vi "FeedbackDecode_20200902.vi"() -> ()   [LabVIEW 2016] (continued)
                n759 = Format Into String(w469) -> (resulting string=w459:string)  [unwired: 3 in, 1 out]
                n760 = Concatenate Strings("ExcludeSE:SS.EventID=" ("string"), w459) -> (w468:string)
                n761 = call-poly "FeedbackDecode_VariablesToString.vi"("Format"="%0.0f", "ValueIn"=w463, "FieldName"="NIPTime" ("Key Word")) -> ("StringOut"=w460:string)  [unwired: 4 in]
                n762 = local read "EventParamsFID"() -> (w466:refnum<file>)
                n763 = local read "DecodeClust"() -> (w472:T5)
                n764 = Concatenate Strings(w468, ";SS.ExcludeSE=1;" ("EventStr"), w460) -> (w465:string)
                n765 = call "FeedbackDecode_WriteTextEOL.vi"("text"=w465, "refnum in"=w466) -> ()  [unwired: 8 in, 2 out]
                n766 = Bundle By Name(cluster=w472, "EventStr"=w465) -> (w464:T5)
                n767 = call "FeedbackDecode_MLComCtrl.vi"("DecodeClustIn"=w464, "Mode"=T19."SendEvent") -> ()  [unwired: 6 in, 4 out]
              }
            }
          }
          event Value Change {
            n768 = event-data() -> ("NewVal"=w474:bool)  [unwired: 1 in, 5 out]
            n769 = case shown="True" w474 {
              frame False {
                n770 = local read "LoopCnt"() -> (w485:u64)
                n771 = local read "NIPTime"() -> (w479:dbl)
                n772 = Format Into String(w485) -> (resulting string=w475:string)  [unwired: 3 in, 1 out]
                n773 = Concatenate Strings("StopAcqCAR:SS.EventID=" ("string"), w475) -> (w484:string)
                n774 = local read "EventParamsFID"() -> (w482:refnum<file>)
                n775 = call-poly "FeedbackDecode_VariablesToString.vi"("Format"="%0.0f", "ValueIn"=w479, "FieldName"="NIPTime" ("Key Word")) -> ("StringOut"=w476:string)  [unwired: 4 in]
                n776 = local read "DecodeClust"() -> (w488:T5)
                n777 = Concatenate Strings(w484, ";SS.AcqCAR=0;" ("EventStr"), w476) -> (w481:string)
                n778 = call "FeedbackDecode_WriteTextEOL.vi"("text"=w481, "refnum in"=w482) -> ()  [unwired: 8 in, 2 out]
                n779 = Bundle By Name(cluster=w488, "EventStr"=w481) -> (w480:T5)
                n780 = call "FeedbackDecode_MLComCtrl.vi"("DecodeClustIn"=w480, "Mode"=T19."SendEvent") -> ()  [unwired: 6 in, 4 out]
              }
              frame True {
                n781 = local read "LoopCnt"() -> (w499:u64)
                n782 = local read "NIPTime"() -> (w493:dbl)
                n783 = Format Into String(w499) -> (resulting string=w489:string)  [unwired: 3 in, 1 out]
                n784 = call-poly "FeedbackDecode_VariablesToString.vi"("Format"="%0.0f", "ValueIn"=w493, "FieldName"="NIPTime" ("Key Word")) -> ("StringOut"=w490:string)  [unwired: 4 in]
                n785 = Concatenate Strings("StartAcqCAR:SS.EventID=" ("string"), w489) -> (w498:string)
                n786 = local read "EventParamsFID"() -> (w496:refnum<file>)
                n787 = local read "DecodeClust"() -> (w502:T5)
                n788 = Concatenate Strings(w498, ";SS.AcqCAR=1;" ("EventStr"), w490) -> (w495:string)
                n789 = call "FeedbackDecode_WriteTextEOL.vi"("text"=w495, "refnum in"=w496) -> ()  [unwired: 8 in, 2 out]
                n790 = Bundle By Name(cluster=w502, "EventStr"=w495) -> (w494:T5)
                n791 = call "FeedbackDecode_MLComCtrl.vi"("DecodeClustIn"=w494, "Mode"=T19."SendEvent") -> ()  [unwired: 6 in, 4 out]
              }
            }
          }
          event Value Change {
            n792 = event-data() -> ("NewVal"=w504:bool)  [unwired: 1 in, 5 out]
            n793 = case shown="True" w504 {
              frame False {
              }
              frame True {
                n794 = stacked-sequence {
                  frame #0 {
                    n795 = local read "DecodeClust"() -> (w522:T5)
                    n796 = call "FeedbackDecode_MLComCtrl.vi"("DecodeClustIn"=w522, "Mode"=T19."BuildKalmanStr") -> ("DecodeClustOut"=w521:T5)  [unwired: 6 in, 3 out]
                    n797 = Unbundle By Name(w521) -> ("EventStr"=w529:string, "KalmanType"=w510:T44, "KDFFile"=w514:string)
                    n798 = local read "LoopCnt"() -> (w525:u64)
                    n799 = local read "NIPTime"() -> (w519:dbl)
                    n800 = Format Into String(format string="%s", w510) -> (resulting string=w507:string)  [unwired: 2 in, 1 out]
                    n801 = Format Into String(w525) -> (resulting string=w505:string)  [unwired: 3 in, 1 out]
                    n802 = call-poly "FeedbackDecode_VariablesToString.vi"("ValueIn"=w514, "FieldName"="KDFFile") -> ("StringOut"=w513:string)  [unwired: 5 in]
                    n803 = call-poly "FeedbackDecode_VariablesToString.vi"("Format"="%0.0f", "ValueIn"=w519, "FieldName"="NIPTime" ("Key Word")) -> ("StringOut"=w512:string)  [unwired: 4 in]
                    n804 = Concatenate Strings("ApplyTraining:SS.EventID=" ("string"), w505) -> (w524:string)
                    n805 = Concatenate Strings(w524, ";", w529) -> (w516:string)
                    n806 = local read "EventParamsFID"() -> (w523:refnum<file>)
                    n807 = Bundle By Name(cluster=w521, "EventStr"=w516) -> (w520:T5)
                    n808 = Concatenate Strings(w516, "SS.DecodeType='" ("FieldName"), w507, "';" ("string"), w513, w512) -> (w511:string)
                    n809 = call "FeedbackDecode_WriteTextEOL.vi"("text"=w511, "refnum in"=w523) -> ()  [unwired: 8 in, 2 out]
                    n810 = call "FeedbackDecode_MLComCtrl.vi"("DecodeClustIn"=w520, "Mode"=T19."SendEvent") -> ()  [unwired: 6 in, 4 out]
                  }
                  frame #1 {
                    n811 = property on="KinSrc" class="Enum (strict)"("Val(Sgnl)"=enum16{"Off", "Training", "Decode", "COB"}."Decode" ("Value (Signaling)")) -> ()  [unwired: 2 in, 2 out]
                  }
                }
              }
            }
          }
          event Value Change {
            n812 = event-data() -> ("NewVal"=w532:bool)  [unwired: 1 in, 5 out]
            n813 = case shown="True" w532 {
              frame False {
                n814 = local read "LoopCnt"() -> (w544:u64)
                n815 = local read "NIPTime"() -> (w538:dbl)
                n816 = Format Into String(w544) -> (resulting string=w534:string)  [unwired: 3 in, 1 out]
                n817 = call-poly "FeedbackDecode_VariablesToString.vi"("Format"="%0.0f", "ValueIn"=w538, "FieldName"="NIPTime" ("Key Word")) -> ("StringOut"=w535:string)  [unwired: 4 in]
                n818 = Concatenate Strings("DisableBaseline:SS.EventID=" ("string"), w534) -> (w543:string)
                n819 = local read "EventParamsFID"() -> (w541:refnum<file>)
                n820 = local read "DecodeClust"() -> (w547:T5)
                n821 = Concatenate Strings(w543, ";SS.ApplyBaseline=0;" ("EventStr"), w535) -> (w540:string)
                n822 = call "FeedbackDecode_WriteTextEOL.vi"("text"=w540, "refnum in"=w541) -> ()  [unwired: 8 in, 2 out]
                n823 = Bundle By Name(cluster=w547, "EventStr"=w540) -> (w539:T5)
                n824 = call "FeedbackDecode_MLComCtrl.vi"("DecodeClustIn"=w539, "Mode"=T19."SendEvent") -> ()  [unwired: 6 in, 4 out]
              }
              frame True {
                n825 = local read "LoopCnt"() -> (w558:u64)
                n826 = local read "NIPTime"() -> (w552:dbl)
                n827 = Format Into String(w558) -> (resulting string=w548:string)  [unwired: 3 in, 1 out]
                n828 = Concatenate Strings("EnableBaseline:SS.EventID=" ("string"), w548) -> (w557:string)
                n829 = local read "EventParamsFID"() -> (w555:refnum<file>)
                n830 = call-poly "FeedbackDecode_VariablesToString.vi"("Format"="%0.0f", "ValueIn"=w552, "FieldName"="NIPTime" ("Key Word")) -> ("StringOut"=w549:string)  [unwired: 4 in]
                n831 = local read "DecodeClust"() -> (w561:T5)
                n832 = Concatenate Strings(w557, ";SS.ApplyBaseline=1;" ("EventStr"), w549) -> (w554:string)
                n833 = call "FeedbackDecode_WriteTextEOL.vi"("text"=w554, "refnum in"=w555) -> ()  [unwired: 8 in, 2 out]
                n834 = Bundle By Name(cluster=w561, "EventStr"=w554) -> (w553:T5)
                n835 = call "FeedbackDecode_MLComCtrl.vi"("DecodeClustIn"=w553, "Mode"=T19."SendEvent") -> ()  [unwired: 6 in, 4 out]
              }
            }
          }
          event Value Change {
            n836 = event-data() -> ("NewVal"=w562:bool)  [unwired: 1 in, 5 out]
            n837 = case shown="True" w562 {
              frame False {
                n838 = disable-structure shown="Disabled" {
                  frame Disabled {
                    n839 = local read "LoopCnt"() -> (w574:u64)
                    n840 = local read "NIPTime"() -> (w568:dbl)
                    n841 = Format Into String(w574) -> (resulting string=w564:string)  [unwired: 3 in, 1 out]
                    n842 = call-poly "FeedbackDecode_VariablesToString.vi"("Format"="%0.0f", "ValueIn"=w568, "FieldName"="NIPTime" ("Key Word")) -> ("StringOut"=w565:string)  [unwired: 4 in]
                    n843 = Concatenate Strings("DisableBaseline:SS.EventID=" ("string"), w564) -> (w573:string)
                    n844 = local read "EventParamsFID"() -> (w571:refnum<file>)
                    n845 = local read "DecodeClust"() -> (w577:T5)
                    n846 = Concatenate Strings(w573, ";SS.ApplyBaseline=0;" ("EventStr"), w565) -> (w570:string)
                    n847 = call "FeedbackDecode_WriteTextEOL.vi"("text"=w570, "refnum in"=w571) -> ()  [unwired: 8 in, 2 out]
                    n848 = Bundle By Name(cluster=w577, "EventStr"=w570) -> (w569:T5)
                    n849 = call "FeedbackDecode_MLComCtrl.vi"("DecodeClustIn"=w569, "Mode"=T19."SendEvent") -> ()  [unwired: 6 in, 4 out]
                  }
                  frame Enabled {
                  }
                }
              }
              frame True {
                n850 = local read "LoopCnt"() -> (w588:u64)
                n851 = local read "NIPTime"() -> (w582:dbl)
                n852 = Format Into String(w588) -> (resulting string=w578:string)  [unwired: 3 in, 1 out]
                n853 = Concatenate Strings("ExportTraining:SS.EventID=" ("string"), w578) -> (w587:string)
                n854 = local read "EventParamsFID"() -> (w585:refnum<file>)
                n855 = call-poly "FeedbackDecode_VariablesToString.vi"("Format"="%0.0f", "ValueIn"=w582, "FieldName"="NIPTime" ("Key Word")) -> ("StringOut"=w579:string)  [unwired: 4 in]
                n856 = local read "DecodeClust"() -> (w591:T5)
                n857 = Concatenate Strings(w587, ";SS.ExportTraining=1;" ("EventStr"), w579) -> (w584:string)
                n858 = call "FeedbackDecode_WriteTextEOL.vi"("text"=w584, "refnum in"=w585) -> ()  [unwired: 8 in, 2 out]
                n859 = Bundle By Name(cluster=w591, "EventStr"=w584) -> (w583:T5)
                n860 = call "FeedbackDecode_MLComCtrl.vi"("DecodeClustIn"=w583, "Mode"=T19."SendEvent") -> ()  [unwired: 6 in, 4 out]
              }
            }
          }
          event Value Change {
            n861 = event-data() -> ("NewVal"=w592:bool)  [unwired: 1 in, 5 out]
            n862 = case shown="True" w592 {
              frame False {
                n863 = local read "LoopCnt"() -> (w604:u64)
                n864 = local read "NIPTime"() -> (w598:dbl)
                n865 = Format Into String(w604) -> (resulting string=w594:string)  [unwired: 3 in, 1 out]
                n866 = call-poly "FeedbackDecode_VariablesToString.vi"("Format"="%0.0f", "ValueIn"=w598, "FieldName"="NIPTime" ("Key Word")) -> ("StringOut"=w595:string)  [unwired: 4 in]
                n867 = Concatenate Strings("LatchingFilter:SS.EventID=" ("string"), w594) -> (w603:string)
                n868 = local read "EventParamsFID"() -> (w601:refnum<file>)
                n869 = local read "DecodeClust"() -> (w607:T5)
                n870 = Concatenate Strings(w603, ";SS.LatchingFilter=0;" ("EventStr"), w595) -> (w600:string)
                n871 = call "FeedbackDecode_WriteTextEOL.vi"("text"=w600, "refnum in"=w601) -> ()  [unwired: 8 in, 2 out]
                n872 = Bundle By Name(cluster=w607, "EventStr"=w600) -> (w599:T5)
                n873 = call "FeedbackDecode_MLComCtrl.vi"("DecodeClustIn"=w599, "Mode"=T19."SendEvent") -> ()  [unwired: 6 in, 4 out]
              }
              frame True {
                n874 = local read "LoopCnt"() -> (w618:u64)
                n875 = local read "NIPTime"() -> (w612:dbl)
                n876 = Format Into String(w618) -> (resulting string=w608:string)  [unwired: 3 in, 1 out]
                n877 = Concatenate Strings("LatchingFilter:SS.EventID=" ("string"), w608) -> (w617:string)
                n878 = local read "EventParamsFID"() -> (w615:refnum<file>)
                n879 = call-poly "FeedbackDecode_VariablesToString.vi"("Format"="%0.0f", "ValueIn"=w612, "FieldName"="NIPTime" ("Key Word")) -> ("StringOut"=w609:string)  [unwired: 4 in]
                n880 = local read "DecodeClust"() -> (w621:T5)
                n881 = Concatenate Strings(w617, ";SS.LatchingFilter=1;" ("EventStr"), w609) -> (w614:string)
                n882 = call "FeedbackDecode_WriteTextEOL.vi"("text"=w614, "refnum in"=w615) -> ()  [unwired: 8 in, 2 out]
                n883 = Bundle By Name(cluster=w621, "EventStr"=w614) -> (w613:T5)
                n884 = call "FeedbackDecode_MLComCtrl.vi"("DecodeClustIn"=w613, "Mode"=T19."SendEvent") -> ()  [unwired: 6 in, 4 out]
              }
            }
          }
          event Value Change {
            n885 = event-data() -> ("NewVal"=w622:bool)  [unwired: 1 in, 5 out]
            n886 = case shown="True" w622 {
              frame False {
                n887 = local read "LoopCnt"() -> (w634:u64)
                n888 = local read "NIPTime"() -> (w628:dbl)
                n889 = Format Into String(w634) -> (resulting string=w624:string)  [unwired: 3 in, 1 out]
                n890 = call-poly "FeedbackDecode_VariablesToString.vi"("Format"="%0.0f", "ValueIn"=w628, "FieldName"="NIPTime" ("Key Word")) -> ("StringOut"=w625:string)  [unwired: 4 in]
                n891 = Concatenate Strings("EEGTrigger:SS.EventID=" ("string"), w624) -> (w633:string)
                n892 = local read "EventParamsFID"() -> (w631:refnum<file>)
                n893 = local read "DecodeClust"() -> (w637:T5)
                n894 = Concatenate Strings(w633, ";SS.EEGTrigger=0;" ("EventStr"), w625) -> (w630:string)
                n895 = call "FeedbackDecode_WriteTextEOL.vi"("text"=w630, "refnum in"=w631) -> ()  [unwired: 8 in, 2 out]
                n896 = Bundle By Name(cluster=w637, "EventStr"=w630) -> (w629:T5)
                n897 = call "FeedbackDecode_MLComCtrl.vi"("DecodeClustIn"=w629, "Mode"=T19."SendEvent") -> ()  [unwired: 6 in, 4 out]
              }
              frame True {
                n898 = local read "LoopCnt"() -> (w648:u64)
                n899 = local read "NIPTime"() -> (w642:dbl)
                n900 = Format Into String(w648) -> (resulting string=w638:string)  [unwired: 3 in, 1 out]
                n901 = Concatenate Strings("EEGTrigger:SS.EventID=" ("string"), w638) -> (w647:string)
                n902 = local read "EventParamsFID"() -> (w645:refnum<file>)
                n903 = call-poly "FeedbackDecode_VariablesToString.vi"("Format"="%0.0f", "ValueIn"=w642, "FieldName"="NIPTime" ("Key Word")) -> ("StringOut"=w639:string)  [unwired: 4 in]
                n904 = local read "DecodeClust"() -> (w651:T5)
                n905 = Concatenate Strings(w647, ";SS.EEGTrigger=1;" ("EventStr"), w639) -> (w644:string)
                n906 = call "FeedbackDecode_WriteTextEOL.vi"("text"=w644, "refnum in"=w645) -> ()  [unwired: 8 in, 2 out]
                n907 = Bundle By Name(cluster=w651, "EventStr"=w644) -> (w643:T5)
                n908 = call "FeedbackDecode_MLComCtrl.vi"("DecodeClustIn"=w643, "Mode"=T19."SendEvent") -> ()  [unwired: 6 in, 4 out]
              }
            }
          }
          event Value Change {
            n909 = event-data() -> ("NewVal"=w652:bool)  [unwired: 1 in, 5 out]
            n910 = case shown="True" w652 {
              frame False {
                n911 = local read "LoopCnt"() -> (w664:u64)
                n912 = local read "NIPTime"() -> (w658:dbl)
                n913 = Format Into String(w664) -> (resulting string=w654:string)  [unwired: 3 in, 1 out]
                n914 = call-poly "FeedbackDecode_VariablesToString.vi"("Format"="%0.0f", "ValueIn"=w658, "FieldName"="NIPTime" ("Key Word")) -> ("StringOut"=w655:string)  [unwired: 4 in]
                n915 = Concatenate Strings("ConnectECG:SS.EventID=" ("string"), w654) -> (w663:string)
                n916 = local read "EventParamsFID"() -> (w661:refnum<file>)
                n917 = local read "DecodeClust"() -> (w667:T5)
                n918 = Concatenate Strings(w663, ";SS.ConnectECG=0;" ("EventStr"), w655) -> (w660:string)
                n919 = call "FeedbackDecode_WriteTextEOL.vi"("text"=w660, "refnum in"=w661) -> ()  [unwired: 8 in, 2 out]
                n920 = Bundle By Name(cluster=w667, "EventStr"=w660) -> (w659:T5)
                n921 = call "FeedbackDecode_MLComCtrl.vi"("DecodeClustIn"=w659, "Mode"=T19."SendEvent") -> ()  [unwired: 6 in, 4 out]
              }
              frame True {
                n922 = local read "LoopCnt"() -> (w678:u64)
                n923 = local read "NIPTime"() -> (w672:dbl)
                n924 = Format Into String(w678) -> (resulting string=w668:string)  [unwired: 3 in, 1 out]
                n925 = Concatenate Strings("ConnectECG:SS.EventID=" ("string"), w668) -> (w677:string)
                n926 = local read "EventParamsFID"() -> (w675:refnum<file>)
                n927 = call-poly "FeedbackDecode_VariablesToString.vi"("Format"="%0.0f", "ValueIn"=w672, "FieldName"="NIPTime" ("Key Word")) -> ("StringOut"=w669:string)  [unwired: 4 in]
                n928 = local read "DecodeClust"() -> (w681:T5)
                n929 = Concatenate Strings(w677, ";SS.ConnectECG=1;" ("EventStr"), w669) -> (w674:string)
                n930 = call "FeedbackDecode_WriteTextEOL.vi"("text"=w674, "refnum in"=w675) -> ()  [unwired: 8 in, 2 out]
                n931 = Bundle By Name(cluster=w681, "EventStr"=w674) -> (w673:T5)
                n932 = call "FeedbackDecode_MLComCtrl.vi"("DecodeClustIn"=w673, "Mode"=T19."SendEvent") -> ()  [unwired: 6 in, 4 out]
              }
            }
          }
          event Value Change {
            n933 = event-data() -> ("NewVal"=w682:bool)  [unwired: 1 in, 5 out]
            n934 = case shown="True" w682 {
              frame False {
                n935 = local read "LoopCnt"() -> (w694:u64)
                n936 = local read "NIPTime"() -> (w688:dbl)
                n937 = Format Into String(w694) -> (resulting string=w684:string)  [unwired: 3 in, 1 out]
                n938 = call-poly "FeedbackDecode_VariablesToString.vi"("Format"="%0.0f", "ValueIn"=w688, "FieldName"="NIPTime" ("Key Word")) -> ("StringOut"=w685:string)  [unwired: 4 in]
                n939 = Concatenate Strings("ECGTriggerTargets:SS.EventID=" ("string"), w684) -> (w693:string)
                n940 = local read "EventParamsFID"() -> (w691:refnum<file>)
                n941 = local read "DecodeClust"() -> (w697:T5)
                n942 = Concatenate Strings(w693, ";SS.ECGTriggerTargets=0;" ("EventStr"), w685) -> (w690:string)
                n943 = call "FeedbackDecode_WriteTextEOL.vi"("text"=w690, "refnum in"=w691) -> ()  [unwired: 8 in, 2 out]
                n944 = Bundle By Name(cluster=w697, "EventStr"=w690) -> (w689:T5)
                n945 = call "FeedbackDecode_MLComCtrl.vi"("DecodeClustIn"=w689, "Mode"=T19."SendEvent") -> ()  [unwired: 6 in, 4 out]
              }
              frame True {
                n946 = local read "LoopCnt"() -> (w708:u64)
                n947 = local read "NIPTime"() -> (w702:dbl)
                n948 = Format Into String(w708) -> (resulting string=w698:string)  [unwired: 3 in, 1 out]
                n949 = Concatenate Strings("ECGTriggerTargets:SS.EventID=" ("string"), w698) -> (w707:string)
                n950 = local read "EventParamsFID"() -> (w705:refnum<file>)
                n951 = call-poly "FeedbackDecode_VariablesToString.vi"("Format"="%0.0f", "ValueIn"=w702, "FieldName"="NIPTime" ("Key Word")) -> ("StringOut"=w699:string)  [unwired: 4 in]
                n952 = local read "DecodeClust"() -> (w711:T5)
                n953 = Concatenate Strings(w707, ";SS.ECGTriggerTargets=1;" ("EventStr"), w699) -> (w704:string)
                n954 = call "FeedbackDecode_WriteTextEOL.vi"("text"=w704, "refnum in"=w705) -> ()  [unwired: 8 in, 2 out]
                n955 = Bundle By Name(cluster=w711, "EventStr"=w704) -> (w703:T5)
                n956 = call "FeedbackDecode_MLComCtrl.vi"("DecodeClustIn"=w703, "Mode"=T19."SendEvent") -> ()  [unwired: 6 in, 4 out]
              }
            }
          }
          event Value Change {
            n957 = event-data() -> ("NewVal"=w712:bool)  [unwired: 1 in, 5 out]
            n958 = case shown="True" w712 {
              frame False {
                n959 = local read "LoopCnt"() -> (w724:u64)
                n960 = local read "NIPTime"() -> (w718:dbl)
                n961 = Format Into String(w724) -> (resulting string=w714:string)  [unwired: 3 in, 1 out]
                n962 = call-poly "FeedbackDecode_VariablesToString.vi"("Format"="%0.0f", "ValueIn"=w718, "FieldName"="NIPTime" ("Key Word")) -> ("StringOut"=w715:string)  [unwired: 4 in]
                n963 = Concatenate Strings("SecondaryTask:SS.EventID=" ("string"), w714) -> (w723:string)
                n964 = local read "EventParamsFID"() -> (w721:refnum<file>)
                n965 = local read "DecodeClust"() -> (w727:T5)
                n966 = Concatenate Strings(w723, ";SS.SecondaryTask=0;" ("EventStr"), w715) -> (w720:string)
                n967 = call "FeedbackDecode_WriteTextEOL.vi"("text"=w720, "refnum in"=w721) -> ()  [unwired: 8 in, 2 out]
                n968 = Bundle By Name(cluster=w727, "EventStr"=w720) -> (w719:T5)
                n969 = call "FeedbackDecode_MLComCtrl.vi"("DecodeClustIn"=w719, "Mode"=T19."SendEvent") -> ()  [unwired: 6 in, 4 out]
              }
              frame True {
                n970 = local read "LoopCnt"() -> (w738:u64)
                n971 = local read "NIPTime"() -> (w732:dbl)
                n972 = Format Into String(w738) -> (resulting string=w728:string)  [unwired: 3 in, 1 out]
                n973 = Concatenate Strings("SecondaryTask:SS.EventID=" ("string"), w728) -> (w737:string)
                n974 = local read "EventParamsFID"() -> (w735:refnum<file>)
                n975 = call-poly "FeedbackDecode_VariablesToString.vi"("Format"="%0.0f", "ValueIn"=w732, "FieldName"="NIPTime" ("Key Word")) -> ("StringOut"=w729:string)  [unwired: 4 in]
                n976 = local read "DecodeClust"() -> (w741:T5)
                n977 = Concatenate Strings(w737, ";SS.SecondaryTask=1;" ("EventStr"), w729) -> (w734:string)
                n978 = call "FeedbackDecode_WriteTextEOL.vi"("text"=w734, "refnum in"=w735) -> ()  [unwired: 8 in, 2 out]
                n979 = Bundle By Name(cluster=w741, "EventStr"=w734) -> (w733:T5)
                n980 = call "FeedbackDecode_MLComCtrl.vi"("DecodeClustIn"=w733, "Mode"=T19."SendEvent") -> ()  [unwired: 6 in, 4 out]
              }
            }
          }
          event Value Change {
            n981 = event-data() -> ("NewVal"=w745:dbl)  [unwired: 1 in, 5 out]
            n982 = local read "LoopCnt"() -> (w749:u64)
            n983 = local read "NIPTime"() -> (w754:dbl)
            n984 = Format Into String(w749) -> (resulting string=w757:string)  [unwired: 3 in, 1 out]
            n985 = call-poly "FeedbackDecode_VariablesToString.vi"("Format"="%0.0f" ("EventStr"), "ValueIn"=w745, "FieldName"="SecondaryTaskMinBetweenStim" ("EventStr")) -> ("StringOut"=w743:string)  [unwired: 4 in]
            n986 = Concatenate Strings("SecondaryTaskMinBetweenStim:SS.EventID=" ("string"), w757) -> (w750:string)
            n987 = local read "EventParamsFID"() -> (w751:refnum<file>)
            n988 = call-poly "FeedbackDecode_VariablesToString.vi"("Format"="%0.0f", "ValueIn"=w754, "FieldName"="NIPTime" ("Key Word")) -> ("StringOut"=w744:string)  [unwired: 4 in]
            n989 = local read "DecodeClust"() -> (w746:T5)
            n990 = Concatenate Strings(w750, ";" ("EventStr"), w743, w744) -> (w752:string)
            n991 = call "FeedbackDecode_WriteTextEOL.vi"("text"=w752, "refnum in"=w751) -> ()  [unwired: 8 in, 2 out]
            n992 = Bundle By Name(cluster=w746, "EventStr"=w752) -> (w753:T5)
            n993 = call "FeedbackDecode_MLComCtrl.vi"("DecodeClustIn"=w753, "Mode"=T19."SendEvent") -> ()  [unwired: 6 in, 4 out]
          }
          event Value Change {
            n994 = event-data() -> ("NewVal"=w763:dbl)  [unwired: 1 in, 5 out]
            n995 = local read "LoopCnt"() -> (w770:u64)
            n996 = call-poly "FeedbackDecode_VariablesToString.vi"("Format"="%0.0f" ("EventStr"), "ValueIn"=w763, "FieldName"="SecondaryTaskVarBetweenStim" ("EventStr")) -> ("StringOut"=w762:string)  [unwired: 4 in]
            n997 = local read "NIPTime"() -> (w775:dbl)
            n998 = Format Into String(w770) -> (resulting string=w778:string)  [unwired: 3 in, 1 out]
            n999 = Concatenate Strings("SecondaryTaskVarBetweenStim:SS.EventID=" ("string"), w778) -> (w771:string)
            n1000 = local read "EventParamsFID"() -> (w772:refnum<file>)
            n1001 = call-poly "FeedbackDecode_VariablesToString.vi"("Format"="%0.0f", "ValueIn"=w775, "FieldName"="NIPTime" ("Key Word")) -> ("StringOut"=w761:string)  [unwired: 4 in]
            n1002 = local read "DecodeClust"() -> (w767:T5)
            n1003 = Concatenate Strings(w771, ";" ("EventStr"), w762, w761) -> (w773:string)
            n1004 = call "FeedbackDecode_WriteTextEOL.vi"("text"=w773, "refnum in"=w772) -> ()  [unwired: 8 in, 2 out]
            n1005 = Bundle By Name(cluster=w767, "EventStr"=w773) -> (w774:T5)
            n1006 = call "FeedbackDecode_MLComCtrl.vi"("DecodeClustIn"=w774, "Mode"=T19."SendEvent") -> ()  [unwired: 6 in, 4 out]
          }
          event Value Change {
            n1007 = event-data() -> ("NewVal"=w782:dbl)  [unwired: 1 in, 5 out]
            n1008 = local read "LoopCnt"() -> (w789:u64)
            n1009 = local read "NIPTime"() -> (w794:dbl)
            n1010 = Format Into String(w789) -> (resulting string=w797:string)  [unwired: 3 in, 1 out]
            n1011 = call-poly "FeedbackDecode_VariablesToString.vi"("Format"="%0.0f" ("EventStr"), "ValueIn"=w782, "FieldName"="SecondaryTaskStimDur" ("EventStr")) -> ("StringOut"=w781:string)  [unwired: 4 in]
            n1012 = Concatenate Strings("SecondaryTaskStimDur:SS.EventID=" ("string"), w797) -> (w790:string)
            n1013 = local read "EventParamsFID"() -> (w791:refnum<file>)
            n1014 = call-poly "FeedbackDecode_VariablesToString.vi"("Format"="%0.0f", "ValueIn"=w794, "FieldName"="NIPTime" ("Key Word")) -> ("StringOut"=w780:string)  [unwired: 4 in]
            n1015 = local read "DecodeClust"() -> (w786:T5)
            n1016 = Concatenate Strings(w790, ";" ("EventStr"), w781, w780) -> (w792:string)
            n1017 = call "FeedbackDecode_WriteTextEOL.vi"("text"=w792, "refnum in"=w791) -> ()  [unwired: 8 in, 2 out]
            n1018 = Bundle By Name(cluster=w786, "EventStr"=w792) -> (w793:T5)
            n1019 = call "FeedbackDecode_MLComCtrl.vi"("DecodeClustIn"=w793, "Mode"=T19."SendEvent") -> ()  [unwired: 6 in, 4 out]
          }
          event Value Change {
            n1020 = event-data() -> ("NewVal"=w799:bool)  [unwired: 1 in, 5 out]
            n1021 = case shown="True" w799 {
              frame False {
                n1022 = local read "LoopCnt"() -> (w811:u64)
                n1023 = local read "NIPTime"() -> (w805:dbl)
                n1024 = Format Into String(w811) -> (resulting string=w801:string)  [unwired: 3 in, 1 out]
                n1025 = Concatenate Strings("DisableCAR:SS.EventID=" ("string"), w801) -> (w810:string)
                n1026 = local read "EventParamsFID"() -> (w808:refnum<file>)
                n1027 = call-poly "FeedbackDecode_VariablesToString.vi"("Format"="%0.0f", "ValueIn"=w805, "FieldName"="NIPTime" ("Key Word")) -> ("StringOut"=w802:string)  [unwired: 4 in]
                n1028 = local read "DecodeClust"() -> (w814:T5)
                n1029 = Concatenate Strings(w810, ";SS.CAR=0;" ("EventStr"), w802) -> (w807:string)
                n1030 = call "FeedbackDecode_WriteTextEOL.vi"("text"=w807, "refnum in"=w808) -> ()  [unwired: 8 in, 2 out]
                n1031 = Bundle By Name(cluster=w814, "EventStr"=w807) -> (w806:T5)
                n1032 = call "FeedbackDecode_MLComCtrl.vi"("DecodeClustIn"=w806, "Mode"=T19."SendEvent") -> ()  [unwired: 6 in, 4 out]
              }
              frame True {
                n1033 = local read "DecodeClust"() -> (w821:T5)
                n1034 = local read "NIPTime"() -> (w819:dbl)
                n1035 = Unbundle By Name(w821) -> ("BadUEAElects"=w830:dbl[])
                n1036 = local read "LoopCnt"() -> (w827:u64)
                n1037 = call-poly "FeedbackDecode_VariablesToString.vi"("Format"="%0.0f", "ValueIn"=w819, "FieldName"="NIPTime" ("Key Word")) -> ("StringOut"=w816:string)  [unwired: 4 in]
                n1038 = Format Into String(w827) -> (resulting string=w815:string)  [unwired: 3 in, 1 out]
                n1039 = Concatenate Strings("EnableCAR:SS.EventID=" ("string"), w815) -> (w826:string)
                n1040 = call-poly "FeedbackDecode_VariablesToString.vi"("ValueIn"=w830, "FieldName"="BadUEAElects") -> ("StringOut"=w822:string)  [unwired: 5 in]
                n1041 = local read "EventParamsFID"() -> (w824:refnum<file>)
                n1042 = Concatenate Strings(w826, ";SS.CAR=1;" ("EventStr"), w822, w816) -> (w823:string)
                n1043 = call "FeedbackDecode_WriteTextEOL.vi"("text"=w823, "refnum in"=w824) -> ()  [unwired: 8 in, 2 out]
                n1044 = Bundle By Name(cluster=w821, "EventStr"=w823) -> (w820:T5)
                n1045 = call "FeedbackDecode_MLComCtrl.vi"("DecodeClustIn"=w820, "Mode"=T19."SendEvent") -> ()  [unwired: 6 in, 4 out]
              }
            }
          }
          event Value Change {
            n1046 = event-data() -> ("NewVal"=w832:bool)  [unwired: 1 in, 5 out]
            n1047 = case shown="True" w832 {
              frame False {
              }
              frame True {
                n1048 = local read "DecodeClust"() -> (w840:T5)
                n1049 = local read "DecodeClust"() -> (w855:T5)
                n1050 = Bundle By Name(cluster=w855, "CtrlButtons.DEKARestart"=FALSE) -> (w854:T5)
                n1051 = Unbundle By Name(w840) -> ("*Prosthesis"=w839:enum16{"MaleRight", "MaleLeft"})
                n1052 = local write "DecodeClust"(w854) -> ()
                n1053 = local read "LoopCnt"() -> (w850:u64)
                n1054 = local read "NIPTime"() -> (w845:dbl)
                n1055 = Format Into String(w839) -> (resulting string=w838:string)  [unwired: 3 in, 1 out]
                n1056 = Format Into String(w850) -> (resulting string=w842:string)  [unwired: 3 in, 1 out]
                n1057 = Concatenate Strings("RestartDEKA:SS.EventID=" ("string"), w842, ";" ("string")) -> (w849:string)
                n1058 = Concatenate Strings("SS.Prosthesis='" ("EventStr"), w838, "';" ("string")) -> (w834:string)
                n1059 = call-poly "FeedbackDecode_VariablesToString.vi"("Format"="%0.0f", "ValueIn"=w845, "FieldName"="NIPTime" ("Key Word")) -> ("StringOut"=w835:string)  [unwired: 4 in]
                n1060 = global write "FeedbackDecode_Globals.vi" "FD_DEKARestart"(TRUE ("G_DEKARestart")) -> ()
                n1061 = local read "EventParamsFID"() -> (w848:refnum<file>)
                n1062 = Concatenate Strings(w849, w834, w835) -> (w847:string)
                n1063 = call "FeedbackDecode_WriteTextEOL.vi"("text"=w847, "refnum in"=w848) -> ()  [unwired: 8 in, 2 out]
                n1064 = Bundle By Name(cluster=w840, "EventStr"=w847) -> (w846:T5)
                n1065 = call "FeedbackDecode_MLComCtrl.vi"("DecodeClustIn"=w846, "Mode"=T19."SendEvent") -> ()  [unwired: 6 in, 4 out]
              }
            }
          }
          event Value Change {
            n1066 = event-data() -> ("NewVal"=w857:bool)  [unwired: 1 in, 5 out]
            n1067 = case shown="True" w857 {
              frame False {
              }
              frame True {
                n1068 = local read "DecodeClust"() -> (w875:T5)
                n1069 = Bundle By Name(cluster=w875, "CtrlButtons.CalDEKA"=FALSE ("CtrlButtons.DEKARestart")) -> (w874:T5)
                n1070 = local read "LoopCnt"() -> (w869:u64)
                n1071 = local write "DecodeClust"(w874) -> ()
                n1072 = local read "NIPTime"() -> (w864:dbl)
                n1073 = Format Into String(w869) -> (resulting string=w861:string)  [unwired: 3 in, 1 out]
                n1074 = Concatenate Strings("CalibrateDEKA:SS.EventID=" ("string"), w861, ";" ("string")) -> (w868:string)
                n1075 = call-poly "FeedbackDecode_VariablesToString.vi"("Format"="%0.0f", "ValueIn"=w864, "FieldName"="NIPTime" ("Key Word")) -> ("StringOut"=w860:string)  [unwired: 4 in]
                n1076 = local read "EventParamsFID"() -> (w867:refnum<file>)
                n1077 = local read "DecodeClust"() -> (w872:T5)
                n1078 = Concatenate Strings(w868, w860) -> (w866:string)
                n1079 = call "FeedbackDecode_WriteTextEOL.vi"("text"=w866, "refnum in"=w867) -> ()  [unwired: 8 in, 2 out]
                n1080 = Bundle By Name(cluster=w872, "EventStr"=w866) -> (w865:T5)
                n1081 = call "FeedbackDecode_MLComCtrl.vi"("DecodeClustIn"=w865, "Mode"=T19."SendEvent") -> ()  [unwired: 6 in, 4 out]
              }
            }
          }
          event Value Change {
            n1082 = event-data() -> ("NewVal"=w894:bool)  [unwired: 1 in, 5 out]
            n1083 = case shown="True" w894 {
              tunnel: [0.0 1.0] -> w878
              frame False {
              }
              frame True {
                n1084 = local read "DecodeClust"() -> (w900:T5)
                n1085 = Bundle By Name(cluster=w900, "CtrlButtons.CalDEKA"=FALSE ("CtrlButtons.DEKARestart")) -> (w899:T5)
                n1086 = local write "DecodeClust"(w899) -> ()
              }
            }
            n1087 = call-poly "FeedbackDecode_VariablesToString.vi"("Format"="%d", "ValueIn"=w878, "FieldName"="DEKA.Ready" ("string")) -> ("StringOut"=w876:string)  [unwired: 4 in]
            n1088 = local read "LoopCnt"() -> (w890:u64)
            n1089 = local read "NIPTime"() -> (w885:dbl)
            n1090 = Format Into String(w890) -> (resulting string=w882:string)  [unwired: 3 in, 1 out]
            n1091 = Concatenate Strings("ConnectDEKA:SS.EventID=" ("string"), w882, ";" ("string")) -> (w889:string)
            n1092 = call-poly "FeedbackDecode_VariablesToString.vi"("Format"="%0.0f", "ValueIn"=w885, "FieldName"="NIPTime" ("Key Word")) -> ("StringOut"=w877:string)  [unwired: 4 in]
            n1093 = local read "EventParamsFID"() -> (w888:refnum<file>)
            n1094 = local read "DecodeClust"() -> (w893:T5)
            n1095 = Concatenate Strings(w889, w876, w877) -> (w887:string)
            n1096 = call "FeedbackDecode_WriteTextEOL.vi"("text"=w887, "refnum in"=w888) -> ()  [unwired: 8 in, 2 out]
            n1097 = Bundle By Name(cluster=w893, "EventStr"=w887) -> (w886:T5)
            n1098 = call "FeedbackDecode_MLComCtrl.vi"("DecodeClustIn"=w886, "Mode"=T19."SendEvent") -> ()  [unwired: 6 in, 4 out]
          }
          event Value Change {
            n1099 = event-data() -> ("NewVal"=w901:bool)  [unwired: 1 in, 5 out]
            n1100 = case shown="True" w901 {
              frame False {
                n1101 = local read "LoopCnt"() -> (w913:u64)
                n1102 = local read "NIPTime"() -> (w907:dbl)
                n1103 = Format Into String(w913) -> (resulting string=w903:string)  [unwired: 3 in, 1 out]
                n1104 = Concatenate Strings("DisableLog10:SS.EventID=" ("string"), w903) -> (w912:string)
                n1105 = local read "EventParamsFID"() -> (w910:refnum<file>)
                n1106 = call-poly "FeedbackDecode_VariablesToString.vi"("Format"="%0.0f", "ValueIn"=w907, "FieldName"="NIPTime" ("Key Word")) -> ("StringOut"=w904:string)  [unwired: 4 in]
                n1107 = local read "DecodeClust"() -> (w916:T5)
                n1108 = Concatenate Strings(w912, ";SS.Log10=0;" ("EventStr"), w904) -> (w909:string)
                n1109 = call "FeedbackDecode_WriteTextEOL.vi"("text"=w909, "refnum in"=w910) -> ()  [unwired: 8 in, 2 out]
                n1110 = Bundle By Name(cluster=w916, "EventStr"=w909) -> (w908:T5)
                n1111 = call "FeedbackDecode_MLComCtrl.vi"("DecodeClustIn"=w908, "Mode"=T19."SendEvent") -> ()  [unwired: 6 in, 4 out]
              }
              frame True {
                n1112 = local read "LoopCnt"() -> (w928:u64)
                n1113 = local read "NIPTime"() -> (w921:dbl)
                n1114 = Format Into String(w928) -> (resulting string=w917:string)  [unwired: 3 in, 1 out]
                n1115 = Concatenate Strings("EnableLog10:SS.EventID=" ("string"), w917) -> (w927:string)
                n1116 = local read "EventParamsFID"() -> (w925:refnum<file>)
                n1117 = call-poly "FeedbackDecode_VariablesToString.vi"("Format"="%0.0f", "ValueIn"=w921, "FieldName"="NIPTime" ("Key Word")) -> ("StringOut"=w918:string)  [unwired: 4 in]
                n1118 = local read "DecodeClust"() -> (w923:T5)
                n1119 = Concatenate Strings(w927, ";SS.Log10=1;" ("EventStr"), w918) -> (w924:string)
                n1120 = call "FeedbackDecode_WriteTextEOL.vi"("text"=w924, "refnum in"=w925) -> ()  [unwired: 8 in, 2 out]
                n1121 = Bundle By Name(cluster=w923, "EventStr"=w924) -> (w922:T5)
                n1122 = call "FeedbackDecode_MLComCtrl.vi"("DecodeClustIn"=w922, "Mode"=T19."SendEvent") -> ()  [unwired: 6 in, 4 out]
              }
            }
          }
          event Value Change {
            n1123 = event-data() -> ("NewVal"=w931:bool)  [unwired: 1 in, 5 out]
            n1124 = case shown="True" w931 {
              frame False {
                n1125 = local read "LoopCnt"() -> (w943:u64)
                n1126 = local read "NIPTime"() -> (w937:dbl)
                n1127 = Format Into String(w943) -> (resulting string=w933:string)  [unwired: 3 in, 1 out]
                n1128 = Concatenate Strings("DisableReTrain:SS.EventID=" ("string"), w933) -> (w942:string)
                n1129 = call-poly "FeedbackDecode_VariablesToString.vi"("Format"="%0.0f", "ValueIn"=w937, "FieldName"="NIPTime" ("Key Word")) -> ("StringOut"=w934:string)  [unwired: 4 in]
                n1130 = local read "EventParamsFID"() -> (w940:refnum<file>)
                n1131 = local read "DecodeClust"() -> (w946:T5)
                n1132 = Concatenate Strings(w942, ";SS.ReTrain=0;" ("EventStr"), w934) -> (w939:string)
                n1133 = call "FeedbackDecode_WriteTextEOL.vi"("text"=w939, "refnum in"=w940) -> ()  [unwired: 8 in, 2 out]
                n1134 = Bundle By Name(cluster=w946, "EventStr"=w939) -> (w938:T5)
                n1135 = call "FeedbackDecode_MLComCtrl.vi"("DecodeClustIn"=w938, "Mode"=T19."SendEvent") -> ()  [unwired: 6 in, 4 out]
              }
              frame True {
                n1136 = local read "LoopCnt"() -> (w957:u64)
                n1137 = local read "NIPTime"() -> (w951:dbl)
                n1138 = Format Into String(w957) -> (resulting string=w947:string)  [unwired: 3 in, 1 out]
                n1139 = Concatenate Strings("EnableReTrain:SS.EventID=" ("string"), w947) -> (w956:string)
                n1140 = local read "EventParamsFID"() -> (w954:refnum<file>)
                n1141 = call-poly "FeedbackDecode_VariablesToString.vi"("Format"="%0.0f", "ValueIn"=w951, "FieldName"="NIPTime" ("Key Word")) -> ("StringOut"=w948:string)  [unwired: 4 in]
                n1142 = local read "DecodeClust"() -> (w960:T5)
                n1143 = Concatenate Strings(w956, ";SS.ReTrain=1;" ("EventStr"), w948) -> (w953:string)
                n1144 = call "FeedbackDecode_WriteTextEOL.vi"("text"=w953, "refnum in"=w954) -> ()  [unwired: 8 in, 2 out]
                n1145 = Bundle By Name(cluster=w960, "EventStr"=w953) -> (w952:T5)
                n1146 = call "FeedbackDecode_MLComCtrl.vi"("DecodeClustIn"=w952, "Mode"=T19."SendEvent") -> ()  [unwired: 6 in, 4 out]
              }
            }
          }
          event Value Change {
            n1147 = event-data() -> ("NewVal"=w962:dbl)  [unwired: 1 in, 5 out]
            n1148 = local read "LoopCnt"() -> (w975:u64)
            n1149 = call-poly "FeedbackDecode_VariablesToString.vi"("Format"="%0.5f", "ValueIn"=w962, "FieldName"="FreeParam") -> ("StringOut"=w961:string)  [unwired: 4 in]
            n1150 = local read "NIPTime"() -> (w969:dbl)
            n1151 = Format Into String(w975) -> (resulting string=w965:string)  [unwired: 3 in, 1 out]
            n1152 = Concatenate Strings("UpdateFreeParam:SS.EventID=" ("string"), w965) -> (w974:string)
            n1153 = local read "EventParamsFID"() -> (w972:refnum<file>)
            n1154 = call-poly "FeedbackDecode_VariablesToString.vi"("Format"="%0.0f", "ValueIn"=w969, "FieldName"="NIPTime" ("Key Word")) -> ("StringOut"=w966:string)  [unwired: 4 in]
            n1155 = local read "DecodeClust"() -> (w978:T5)
            n1156 = Concatenate Strings(w974, ";" ("EventStr"), w961, w966) -> (w971:string)
            n1157 = call "FeedbackDecode_WriteTextEOL.vi"("text"=w971, "refnum in"=w972) -> ()  [unwired: 8 in, 2 out]
            n1158 = Bundle By Name(cluster=w978, "EventStr"=w971) -> (w970:T5)
            n1159 = call "FeedbackDecode_MLComCtrl.vi"("DecodeClustIn"=w970, "Mode"=T19."SendEvent") -> ()  [unwired: 6 in, 4 out]
          }
          event Value Change {
            n1160 = event-data() -> ("NewVal"=w981:dbl)  [unwired: 1 in, 5 out]
            n1161 = local read "LoopCnt"() -> (w994:u64)
            n1162 = call-poly "FeedbackDecode_VariablesToString.vi"("Format"="%0.5f", "ValueIn"=w981, "FieldName"="GoalNoise") -> ("StringOut"=w980:string)  [unwired: 4 in]
            n1163 = local read "NIPTime"() -> (w988:dbl)
            n1164 = Format Into String(w994) -> (resulting string=w984:string)  [unwired: 3 in, 1 out]
            n1165 = Concatenate Strings("UpdateGoalNoise:SS.EventID=" ("string"), w984) -> (w993:string)
            n1166 = local read "EventParamsFID"() -> (w991:refnum<file>)
            n1167 = call-poly "FeedbackDecode_VariablesToString.vi"("Format"="%0.0f", "ValueIn"=w988, "FieldName"="NIPTime" ("Key Word")) -> ("StringOut"=w985:string)  [unwired: 4 in]
            n1168 = local read "DecodeClust"() -> (w997:T5)
            n1169 = Concatenate Strings(w993, ";" ("EventStr"), w980, w985) -> (w990:string)
            n1170 = call "FeedbackDecode_WriteTextEOL.vi"("text"=w990, "refnum in"=w991) -> ()  [unwired: 8 in, 2 out]
            n1171 = Bundle By Name(cluster=w997, "EventStr"=w990) -> (w989:T5)
            n1172 = call "FeedbackDecode_MLComCtrl.vi"("DecodeClustIn"=w989, "Mode"=T19."SendEvent") -> ()  [unwired: 6 in, 4 out]
          }
          event "OffSet": Value Change {
            n1173 = event-data() -> ("NewVal"=w1000:dbl)  [unwired: 1 in, 5 out]
            n1174 = global write "FeedbackDecode_Globals.vi" "FD_ForceOffset"(w1000) -> ()
          }
          event Value Change {
            n1175 = event-data() -> ("NewVal"=w1002:bool)  [unwired: 1 in, 5 out]
            n1176 = case shown="True" w1002 {
              frame False {
              }
              frame True {
                n1177 = local read "DecodeClust"() -> (w1007:T5)
                n1178 = Unbundle By Name(w1007) -> ("CompID.ML.Name"=w1006:string, "DataFolder"=w1005:string, "DataDir"=w1003:string, "NumComp"=w1004:enum16{"1 Computer", "2 Computers"})
                n1179 = case shown="\"1 Computer\"" w1004 {
                  tunnel: w1007 -> [w1027 w1056]
                  tunnel: w1006 -> [w1011 _]
                  tunnel: w1005 -> [w1010 w1040]
                  tunnel: w1003 -> [_ w1037]
                  frame "2 Computers", Default {
                    n1180 = call "FeedbackDecode_CopyRemoteFiles.vi"("DataFolder"=w1010, "CompName"=w1011, "Mode"=enum16{"Decode", "Encode"}."Decode") -> ("OrigName"=w1008:string, "MLName"=w1034:string)  [unwired: 1 in]
                    n1181 = local read "LoopCnt"() -> (w1024:u64)
                    n1182 = local read "NIPTime"() -> (w1028:dbl)
                    n1183 = String To Path(string=w1034) -> (path=w1033:path)
                    n1184 = Strip Path(path=w1033) -> (name=w1035:string)  [unwired: 1 out]
                    n1185 = Format Into String(w1024) -> (resulting string=w1036:string)  [unwired: 3 in, 1 out]
                    n1186 = call-poly "FeedbackDecode_VariablesToString.vi"("Format"="%0.0f", "ValueIn"=w1028, "FieldName"="NIPTime" ("Key Word")) -> ("StringOut"=w1031:string)  [unwired: 4 in]
                    n1187 = Concatenate Strings("SS.TrainFileLV='" ("string"), w1034, "';" ("string")) -> (w1018:string)
                    n1188 = Concatenate Strings("LoadTrainFile:SS.EventID=" ("string"), w1036) -> (w1025:string)
                    n1189 = Concatenate Strings("SS.TrainFileOrig='" ("string"), w1008, "';" ("string"), w1031) -> (w1014:string)
                    n1190 = Concatenate Strings(w1025, ";", w1018) -> (w1017:string)
                    n1191 = Concatenate Strings(w1017, w1014) -> (w1012:string)
                    n1192 = Bundle By Name(cluster=w1027, "KDFFile"=w1035, "EventStr"=w1017) -> (w1026:T5)
                    n1193 = local read "EventParamsFID"() -> (w1013:refnum<file>)
                    n1194 = call "FeedbackDecode_WriteTextEOL.vi"("text"=w1012, "refnum in"=w1013) -> ()  [unwired: 8 in, 2 out]
                    n1195 = call "FeedbackDecode_MLComCtrl.vi"("DecodeClustIn"=w1026, "Mode"=T19."SendEvent") -> ("DecodeClustOut"=w1032:T5)  [unwired: 6 in, 3 out]
                    n1196 = local write "DecodeClust"(w1032) -> ()
                  }
                  frame "1 Computer" {
                    n1197 = call "FeedbackDecode_CopyLocalFiles.vi"("DataFolder"=w1040, "DataDir"=w1037, "Mode"=enum16{"Decode", "Encode"}."Decode") -> ("OrigName"=w1038:string, "MLName"=w1063:string)  [unwired: 1 in]
                    n1198 = local read "LoopCnt"() -> (w1053:u64)
                    n1199 = local read "NIPTime"() -> (w1057:dbl)
                    n1200 = String To Path(string=w1063) -> (path=w1062:path)
                    n1201 = Strip Path(path=w1062) -> (name=w1064:string)  [unwired: 1 out]
                    n1202 = Format Into String(w1053) -> (resulting string=w1065:string)  [unwired: 3 in, 1 out]
                    n1203 = call-poly "FeedbackDecode_VariablesToString.vi"("Format"="%0.0f", "ValueIn"=w1057, "FieldName"="NIPTime" ("Key Word")) -> ("StringOut"=w1060:string)  [unwired: 4 in]
                    n1204 = Concatenate Strings("SS.TrainFileLV='" ("string"), w1063, "';" ("string")) -> (w1047:string)
                    n1205 = Concatenate Strings("LoadTrainFile:SS.EventID=" ("string"), w1065) -> (w1054:string)
                    n1206 = Concatenate Strings("SS.TrainFileOrig='" ("string"), w1038, "';" ("string"), w1060) -> (w1043:string)
                    n1207 = Concatenate Strings(w1054, ";", w1047) -> (w1046:string)
                    n1208 = Concatenate Strings(w1046, w1043) -> (w1041:string)
                    n1209 = Bundle By Name(cluster=w1056, "KDFFile"=w1064, "EventStr"=w1046) -> (w1055:T5)
                    n1210 = local read "EventParamsFID"() -> (w1042:refnum<file>)
                    n1211 = call "FeedbackDecode_WriteTextEOL.vi"("text"=w1041, "refnum in"=w1042) -> ()  [unwired: 8 in, 2 out]
                    n1212 = call "FeedbackDecode_MLComCtrl.vi"("DecodeClustIn"=w1055, "Mode"=T19."SendEvent") -> ("DecodeClustOut"=w1061:T5)  [unwired: 6 in, 3 out]
                    n1213 = local write "DecodeClust"(w1061) -> ()
                  }
                }
              }
            }
          }
          event Value Change {
            n1214 = event-data() -> ("NewVal"=w1067:bool)  [unwired: 1 in, 5 out]
            n1215 = case shown="True" w1067 {
              frame False {
                n1216 = local read "LoopCnt"() -> (w1078:u64)
                n1217 = local read "NIPTime"() -> (w1072:dbl)
                n1218 = Format Into String(w1078) -> (resulting string=w1068:string)  [unwired: 3 in, 1 out]
                n1219 = Concatenate Strings("DisableNIPSpikes:SS.EventID=" ("string"), w1068) -> (w1077:string)
                n1220 = local read "EventParamsFID"() -> (w1075:refnum<file>)
                n1221 = call-poly "FeedbackDecode_VariablesToString.vi"("Format"="%0.0f", "ValueIn"=w1072, "FieldName"="NIPTime" ("Key Word")) -> ("StringOut"=w1069:string)  [unwired: 4 in]
                n1222 = local read "DecodeClust"() -> (w1081:T5)
                n1223 = Concatenate Strings(w1077, ";SS.NIPSpikes=0;" ("EventStr"), w1069) -> (w1074:string)
                n1224 = call "FeedbackDecode_WriteTextEOL.vi"("text"=w1074, "refnum in"=w1075) -> ()  [unwired: 8 in, 2 out]
                n1225 = Bundle By Name(cluster=w1081, "EventStr"=w1074) -> (w1073:T5)
                n1226 = call "FeedbackDecode_MLComCtrl.vi"("DecodeClustIn"=w1073, "Mode"=T19."SendEvent") -> ()  [unwired: 6 in, 4 out]
              }
              frame True {
                n1227 = local read "LoopCnt"() -> (w1092:u64)
                n1228 = local read "NIPTime"() -> (w1086:dbl)
                n1229 = Format Into String(w1092) -> (resulting string=w1082:string)  [unwired: 3 in, 1 out]
                n1230 = Concatenate Strings("EnableNIPSpikes:SS.EventID=" ("string"), w1082) -> (w1091:string)
                n1231 = call-poly "FeedbackDecode_VariablesToString.vi"("Format"="%0.0f", "ValueIn"=w1086, "FieldName"="NIPTime" ("Key Word")) -> ("StringOut"=w1083:string)  [unwired: 4 in]
                n1232 = local read "EventParamsFID"() -> (w1089:refnum<file>)
                n1233 = local read "DecodeClust"() -> (w1095:T5)
                n1234 = Concatenate Strings(w1091, ";SS.NIPSpikes=1;" ("EventStr"), w1083) -> (w1088:string)
                n1235 = call "FeedbackDecode_WriteTextEOL.vi"("text"=w1088, "refnum in"=w1089) -> ()  [unwired: 8 in, 2 out]
                n1236 = Bundle By Name(cluster=w1095, "EventStr"=w1088) -> (w1087:T5)
                n1237 = call "FeedbackDecode_MLComCtrl.vi"("DecodeClustIn"=w1087, "Mode"=T19."SendEvent") -> ()  [unwired: 6 in, 4 out]
              }
            }
          }
          event Value Change {
            n1238 = event-data() -> ("NewVal"=w1097:bool)  [unwired: 1 in, 5 out]
            n1239 = case shown="True" w1097 {
              frame False {
              }
              frame True {
                n1240 = local read "DecodeClust"() -> (w1125:T5)
                n1241 = Unbundle By Name(w1125) -> ("AutoPopType"=w1101:enum16{"Standard", "Stepwise", "Gram"}, "AutoThresh"=w1122:dbl, "BadUEAElects"=w1115:dbl[], "BadEMGChans"=w1119:dbl[])
                n1242 = Format Into String(w1101) -> (resulting string=w1099:string)  [unwired: 3 in, 1 out]
                n1243 = local read "LoopCnt"() -> (w1111:u64)
                n1244 = call-poly "FeedbackDecode_VariablesToString.vi"("ValueIn"=w1099, "FieldName"="AutoPopType" ("Key Word")) -> ("StringOut"=w1098:string)  [unwired: 5 in]
                n1245 = call-poly "FeedbackDecode_VariablesToString.vi"("ValueIn"=w1122, "FieldName"="AutoThresh") -> ("StringOut"=w1118:string)  [unwired: 5 in]
                n1246 = call-poly "FeedbackDecode_VariablesToString.vi"("ValueIn"=w1115, "FieldName"="BadUEAElects") -> ("StringOut"=w1117:string)  [unwired: 5 in]
                n1247 = call-poly "FeedbackDecode_VariablesToString.vi"("ValueIn"=w1119, "FieldName"="BadEMGChans") -> ("StringOut"=w1116:string)  [unwired: 5 in]
                n1248 = Format Into String(w1111) -> (resulting string=w1102:string)  [unwired: 3 in, 1 out]
                n1249 = local read "NIPTime"() -> (w1106:dbl)
                n1250 = Concatenate Strings(w1098, w1118, w1117, w1116) -> (w1124:string)
                n1251 = Concatenate Strings("AutoPop:SS.EventID=" ("string"), w1102) -> (w1110:string)
                n1252 = local read "EventParamsFID"() -> (w1109:refnum<file>)
                n1253 = call-poly "FeedbackDecode_VariablesToString.vi"("Format"="%0.0f", "ValueIn"=w1106, "FieldName"="NIPTime" ("Key Word")) -> ("StringOut"=w1103:string)  [unwired: 4 in]
                n1254 = Concatenate Strings(w1110, ";", w1124, w1103) -> (w1108:string)
                n1255 = call "FeedbackDecode_WriteTextEOL.vi"("text"=w1108, "refnum in"=w1109) -> ()  [unwired: 8 in, 2 out]
                n1256 = Bundle By Name(cluster=w1125, "EventStr"=w1108) -> (w1107:T5)
                n1257 = call "FeedbackDecode_MLComCtrl.vi"("DecodeClustIn"=w1107, "Mode"=T19."SendEvent") -> ()  [unwired: 6 in, 4 out]
              }
            }
          }
          event Value Change {
            n1258 = event-data() -> ()  [unwired: 1 in, 6 out]
            n1259 = local read "DecodeClust"() -> (w1146:T5)
            n1260 = Unbundle By Name(w1146) -> ("BadUEAElects"=w1138:dbl[], "BadEMGChans"=w1141:dbl[])
            n1261 = local read "LoopCnt"() -> (w1134:u64)
            n1262 = call-poly "FeedbackDecode_VariablesToString.vi"("ValueIn"=w1138, "FieldName"="BadUEAElects") -> ("StringOut"=w1140:string)  [unwired: 5 in]
            n1263 = call-poly "FeedbackDecode_VariablesToString.vi"("ValueIn"=w1141, "FieldName"="BadEMGChans") -> ("StringOut"=w1139:string)  [unwired: 5 in]
            n1264 = Format Into String(w1134) -> (resulting string=w1126:string)  [unwired: 3 in, 1 out]
            n1265 = local read "NIPTime"() -> (w1130:dbl)
            n1266 = Concatenate Strings(w1140, w1139) -> (w1144:string)
            n1267 = Concatenate Strings("SendBad:SS.EventID=" ("string"), w1126) -> (w1133:string)
            n1268 = local read "EventParamsFID"() -> (w1145:refnum<file>)
            n1269 = call-poly "FeedbackDecode_VariablesToString.vi"("Format"="%0.0f", "ValueIn"=w1130, "FieldName"="NIPTime" ("Key Word")) -> ("StringOut"=w1127:string)  [unwired: 4 in]
            n1270 = Concatenate Strings(w1133, ";", w1144, w1127) -> (w1132:string)
            n1271 = call "FeedbackDecode_WriteTextEOL.vi"("text"=w1132, "refnum in"=w1145) -> ()  [unwired: 8 in, 2 out]
            n1272 = Bundle By Name(cluster=w1146, "EventStr"=w1132) -> (w1131:T5)
            n1273 = call "FeedbackDecode_MLComCtrl.vi"("DecodeClustIn"=w1131, "Mode"=T19."SendEvent") -> ()  [unwired: 6 in, 4 out]
          }
          event Value Change {
            n1274 = event-data() -> ("NewVal"=w1150:bool)  [unwired: 1 in, 5 out]
            n1275 = Not(x=w1150) -> (.not. x?=w1149:bool)
            n1276 = local read "DecodeClust"() -> (w1151:T5)
            n1277 = Bundle By Name(cluster=w1151, "CtrlButtons.Stop"=w1149) -> (w1148:T5)
            n1278 = local write "DecodeClust"(w1148) -> ()
            n1279 = property on="Finished" class="Bool (strict)"("DisabledEnum"=T17."Enabled" ("Disabled"), "Blinking"=TRUE) -> ()  [unwired: 2 in, 2 out]
            n1280 = local write "LVTab"(enum32{"Decode", "Encode", "Video", "Database"}."Database" ("LVTab")) -> ()
          }
          event "Finished": Value Change {
            n1281 = event-data() -> ("NewVal"=w1156:bool)  [unwired: 1 in, 5 out]
            n1282 = global write "FeedbackDecode_Globals.vi" "FD_Stop"(w1156) -> ()
          }
          event Value Change {
            n1283 = event-data() -> ("NewVal"=w1157:bool)  [unwired: 1 in, 5 out]
            n1284 = case shown="True" w1157 {
              frame False {
                n1285 = local read "LoopCnt"() -> (w1167:u64)
                n1286 = local read "NIPTime"() -> (w1163:dbl)
                n1287 = Format Into String(w1167) -> (resulting string=w1159:string)  [unwired: 3 in, 1 out]
                n1288 = local read "EventParamsFID"() -> (w1171:refnum<file>)
                n1289 = local read "DecodeClust"() -> (w1172:T5)
                n1290 = call-poly "FeedbackDecode_VariablesToString.vi"("Format"="%0.0f", "ValueIn"=w1163, "FieldName"="NIPTime" ("Key Word")) -> ("StringOut"=w1160:string)  [unwired: 4 in]
                n1291 = Concatenate Strings("DisableStartTrials:SS.EventID=" ("string"), w1159) -> (w1166:string)
                n1292 = Concatenate Strings(w1166, ";", w1160) -> (w1165:string)
                n1293 = call "FeedbackDecode_WriteTextEOL.vi"("text"=w1165, "refnum in"=w1171) -> ()  [unwired: 8 in, 2 out]
                n1294 = Bundle By Name(cluster=w1172, "EventStr"=w1165) -> (w1164:T5)
                n1295 = call "FeedbackDecode_MLComCtrl.vi"("DecodeClustIn"=w1164, "Mode"=T19."SendEvent") -> ()  [unwired: 6 in, 4 out]
              }
              frame True {
                n1296 = local read "LoopCnt"() -> (w1186:u64)
                n1297 = local read "NIPTime"() -> (w1177:dbl)
                n1298 = Format Into String(w1186) -> (resulting string=w1173:string)  [unwired: 3 in, 1 out]
                n1299 = local read "EventParamsFID"() -> (w1190:refnum<file>)
                n1300 = call-poly "FeedbackDecode_VariablesToString.vi"("Format"="%0.0f", "ValueIn"=w1177, "FieldName"="NIPTime" ("Key Word")) -> ("StringOut"=w1174:string)  [unwired: 4 in]
                n1301 = Concatenate Strings("EnableStartTrials:SS.EventID=" ("string"), w1173) -> (w1185:string)
                n1302 = Concatenate Strings(w1185, ";", w1174) -> (w1184:string)
                n1303 = local read "DecodeClust"() -> (w1191:T5)
